vi "configure.vi"(8 "error in (no error)":errorcluster, 11 "DAQ_DL091205Readers in":refnum<class "DAQ_DL091205Readers.lvclass">) -> (0 "error out":errorcluster, 3 "DAQ_DL091205Readers out":refnum<class "DAQ_DL091205Readers.lvclass">)   [LabVIEW 2010, in "DAQ_DL091205Readers.lvclass"]
doc: "The dynamic dispatch version of this VI loads and displays the configuration file associated with the plug-in object. The user modify and save the configuration data."
uses:
  DAQ_DL091205Readers.lvclass
  DAQ_DL091205Readers.lvclass/DAQ_DL091205Readers.ctl
  SignalReader/GenericSignalReader/GenericSignalReader/GenericSignalReader.lvclass
  common/classes/ErrorController/ErrorController/class_data.vi
  common/classes/GenericComponent/GenericComponent/GenericComponent.lvclass
  common/classes/ErrorController/ErrorController/ErrorController.lvclass
panel:
  in  "software buffer size":i32=16000 min=0
  in  "read block size":i32=16000 min=0
  out "LSID":string
  out "Configuration":string
  in  "editSignalReadersListButton":bool
  in  "cancelButton":bool
  in  "saveButton":bool
  # "Configure DAQ_DL091205Readers"
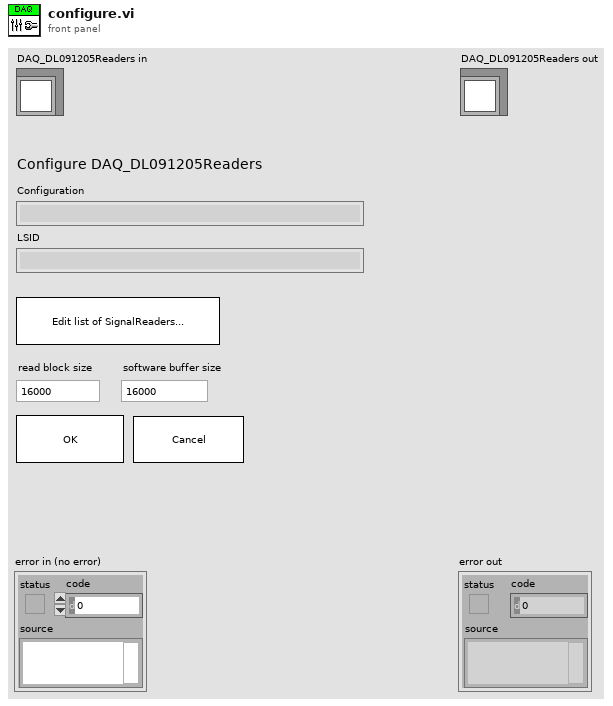
[diagram p1: front panel]
types:
  T1 = typedef "LSID_cluster.ctl" = cluster{"identifier":string, "revision":i32}
  T2 = typedef "DAQ_DL091205Readers.lvclass/config_data_cluster.ctl" = cluster{"readers":T3[], "LSID":T1, "read block size":i32, "software buffer size":i32}
  T3 = typedef "plugin_specification.ctl" = cluster{"class path":string, "configuration":string, "label":string, "settings name":string}
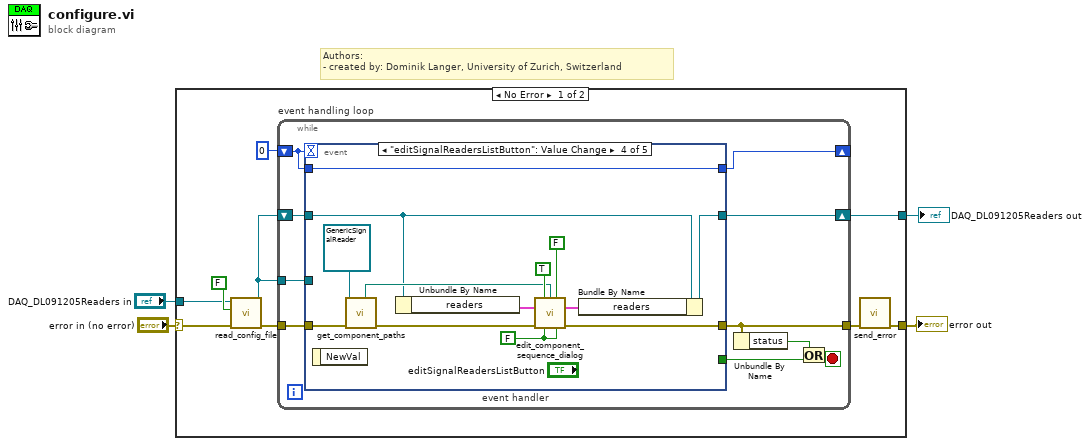
[diagram p0: block diagram]
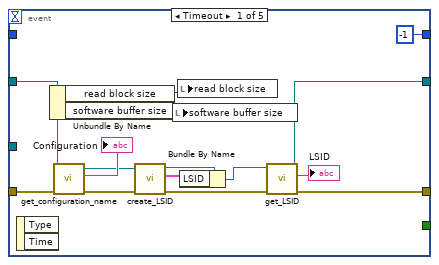
[diagram p2: hidden frame]
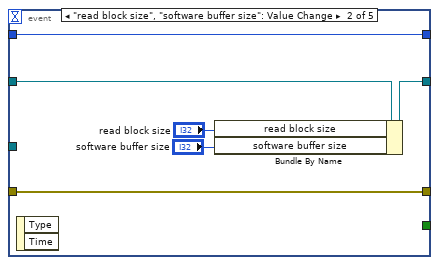
[diagram p3: hidden frame]
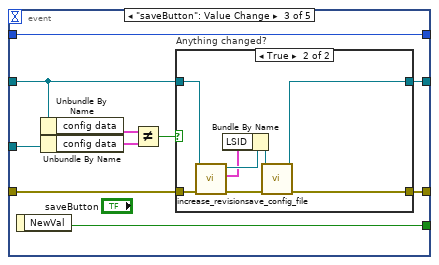
[diagram p4: hidden frame]
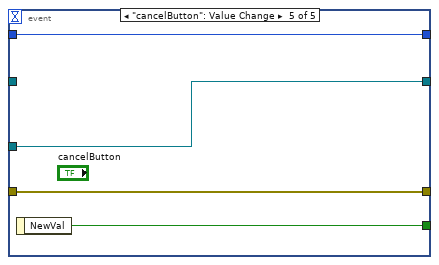
[diagram p6: hidden frame]
diagram:
  # "Authors: \n- created by: Dominik Langer, University of Zurich, Switzerland"
  n1 = case shown="No Error" "error in (no error)" {
    selector: "error in (no error)" -> [w12 w83]
    tunnel: "DAQ_DL091205Readers in" -> [w9 w82]
    tunnel: [w6 w83] -> w2
    tunnel: [w13 w82] -> w1
    frame No Error {
      n2 = call-dynamic "read_config_file.vi"("error in (no error)"=w12, "force load?"=FALSE, "GenericPlugin in"=w9) -> ("error out"=w11:errorcluster, "GenericPlugin out"=w8:refnum<class "DAQ_DL091205Readers.lvclass">)  [unwired: 7 in]
      n3 = while "event handling loop" {
        shift-right: [w21] -> w13
        shift-left: w8 -> [w22]
        tunnel: w8 -> [w20]
        shift-right: [w18] -> _
        shift-left: 0 -> [w19]
        tunnel: w11 -> [w23]
        tunnel: [w17] -> w5
        stop <- w14 stop-if-true
        n4 = event "event handler" shown="[3] \"editSignalReadersListButton\": Value Change" {
          selector: _ -> [_ _ _ _ _]
          dyn-events: _ -> [_ _ _ _ _]
          timeout: w19 -> [_ _ _ _ _]
          tunnel: w23 -> [w38 w44 w53 w68 w81]
          tunnel: w22 -> [w27 w42 w50 w65 _]
          tunnel: [w24 w44 w52 w77 w81] -> w17
          tunnel: [w33 w41 w51 w75 w80] -> w21
          tunnel: w20 -> [_ _ w49 _ w80]
          tunnel: [_ _ w54 _ w79] -> w15
          tunnel: w19 -> [_ w43 w45 w70 w78]
          tunnel: [-1 w43 w45 w70 w78] -> w18
          event Timeout {
            n5 = event-data() -> ()  [unwired: 1 in, 2 out]
            n6 = Unbundle By Name(w27) -> ("read block size"=w25:i32, "software buffer size"=w26:i32)
            n7 = call "get_configuration_name.vi"("error in (no error)"=w38, "GenericPlugin.lvclass in"=w27) -> ("error out"=w36:errorcluster, "configuration name"=→"Configuration":string, "GenericPlugin.lvclass out"=w35:refnum<class "DAQ_DL091205Readers.lvclass">)  [unwired: 7 in]
            n8 = call-dynamic "create_LSID.vi"("error in (no error)"=w36, "GenericPlugin in"=w35) -> ("error out"=w34:errorcluster, "current LSID"=w31:T1, "GenericPlugin out"=w30:refnum<class "DAQ_DL091205Readers.lvclass">)  [unwired: 7 in]
            n9 = local write "software buffer size"(w26) -> ()
            n10 = local write "read block size"(w25) -> ()
            n11 = Bundle By Name(cluster=w30, "LSID"=w31) -> (w29:refnum<class "DAQ_DL091205Readers.lvclass">)
            n12 = call-dynamic "get_LSID.vi"("error in (no error)"=w34, "GenericPlugin in"=w29) -> ("error out"=w24:errorcluster, "LSID (string)"=→"LSID":string, "GenericPlugin out"=w33:refnum<class "DAQ_DL091205Readers.lvclass">)  [unwired: 6 in, 1 out]
          }
          event "read block size", "software buffer size": Value Change {
            n13 = event-data() -> ()  [unwired: 1 in, 2 out]
            n14 = Bundle By Name(cluster=w42, "read block size"="read block size", "software buffer size"="software buffer size") -> (w41:refnum<class "DAQ_DL091205Readers.lvclass">)
          }
          event "saveButton": Value Change {
            n15 = event-data() -> ("NewVal"=w54:bool)  [unwired: 1 in]
            n16 = Unbundle By Name(w50) -> ("config data"=w46:T2)
            n17 = Unbundle By Name(w49) -> ("config data"=w48:T2)
            n18 = Not Equal?(x=w46, y=w48) -> (x != y?=w47:bool)
            n19 = case "Anything changed?" shown="True" w47 {
              tunnel: w53 -> [w55 w62]
              tunnel: [w55 w64] -> w52
              tunnel: [w56 w63] -> w51
              tunnel: w50 -> [w56 w60]
              frame False {
              }
              frame True {
                n20 = call-dynamic "increase_revision.vi"("error in (no error)"=w62, "GenericPlugin in"=w60) -> ("error out"=w61:errorcluster, "new LSID"=w58:T1, "GenericPlugin out"=w59:refnum<class "DAQ_DL091205Readers.lvclass">)  [unwired: 7 in]
                n21 = Bundle By Name(cluster=w59, "LSID"=w58) -> (w57:refnum<class "DAQ_DL091205Readers.lvclass">)
                n22 = call-dynamic "save_config_file.vi"("error in (no error)"=w61, "GenericPlugin in"=w57) -> ("error out"=w64:errorcluster, "GenericPlugin out"=w63:refnum<class "DAQ_DL091205Readers.lvclass">)  [unwired: 8 in]
              }
            }
          }
          event "editSignalReadersListButton": Value Change {
            w71 = FALSE ("choose default?")
            n23 = event-data() -> ()  [unwired: 1 in, 1 out]
            n24 = call-dynamic "get_component_paths.vi"("error in (no error)"=w68, "GenericComponent in"=refnum<class "GenericSignalReader.lvclass"> refnum ("GenericSignalReader.lvclass")) -> ("error out"=w67:errorcluster, "component type directory"=w66:path)  [unwired: 4 in, 4 out]
            n25 = Unbundle By Name(w65) -> ("readers"=w76:T3[])
            n26 = call "edit_component_sequence_dialog.vi"("show configuration?"=TRUE, "default folder path"=w66, "show label?"=FALSE, "component specification list in"=w76, "error in (no error)"=w67, "choose default?"=w71, "show settings?"=w71) -> ("component specification list out"=w74:T3[], "error out"=w77:errorcluster)  [unwired: 6 in, 1 out]
            n27 = Bundle By Name(cluster=w65, "readers"=w74) -> (w75:refnum<class "DAQ_DL091205Readers.lvclass">)
          }
          event "cancelButton": Value Change {
            n28 = event-data() -> ("NewVal"=w79:bool)  [unwired: 1 in]
          }
        }
        n29 = Unbundle By Name(w17) -> ("status"=w16:bool)
        n30 = Or(x=w16, y=w15) -> (x .or. y?=w14:bool)
      }
      n31 = call "send_error.vi"("error in (no error)"=w5) -> ("error out"=w6:errorcluster)  [unwired: 10 in]
    }
    frame Error {
    }
  }
  "error out" <- w2
  "DAQ_DL091205Readers out" <- w1
